vi "Write settings button array for hardware.vi"(8 "error in (no error)":errorcluster, 10 "settings button array for hardware":refnum<vi>[](array[refnum]), 11 "Measurement UI in":refnum<class "Measurement UI.lvclass">) -> (0 "error out":errorcluster, 3 "Measurement UI out":refnum<class "Measurement UI.lvclass">)   [LabVIEW 2016, in "Measurement UI.lvlib" / "Measurement UI.lvclass"]
uses:
  Measurement UI.lvclass
  Measurement UI.lvclass/Measurement UI.ctl
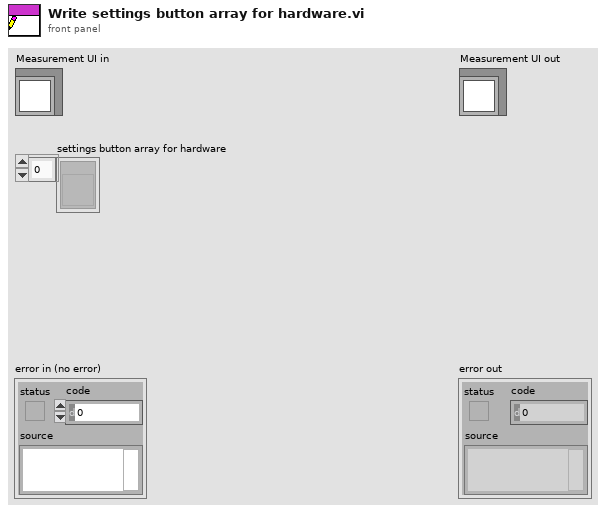
[diagram p1: front panel]
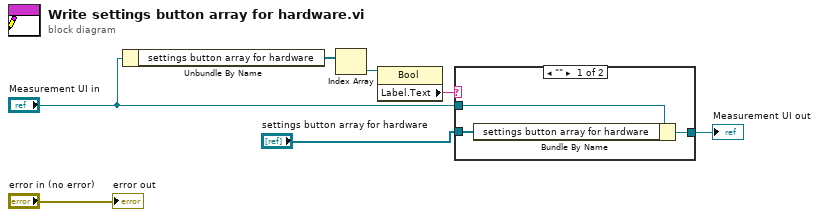
[diagram p0: block diagram]
diagram:
  n1 = Unbundle By Name("Measurement UI in") -> ("settings button array for hardware"=w3:refnum<vi>[])
  n2 = Index Array(array=w3) -> (element=w2:refnum<vi>)  [unwired: 1 in]
  n3 = property class="Bool"(reference=w2) -> ("Label.Text"=w7:string)  [unwired: 1 in, 2 out]
  n4 = case shown="\"\"" w7 {
    tunnel: "Measurement UI in" -> [w9 w11]
    tunnel: "settings button array for hardware" -> [w10 _]
    tunnel: [w8 w11] -> w4
    frame "" {
      n5 = Bundle By Name(cluster=w9, "settings button array for hardware"=w10) -> (w8:refnum<class "Measurement UI.lvclass">)
    }
    frame Default {
    }
  }
  "Measurement UI out" <- w4
  "error out" <- "error in (no error)"
